vi "Shapelets Search (Brute Force).vi"() -> ()   [LabVIEW 2016]
uses:
  <vilib>/Math Plots/3D Math Plots/3D Ribbon/3D Ribbon XCtrl/3D Ribbon.xctl
  _vlib/SH_ApplicationStates.ctl
  _vlib/Shapelets Search Brute Force.lvclass
  _vlib/SH_Shapelet.ctl
  <vilib>/Math Plots/3D Math Plots/3D Ribbon/3D Ribbon Datatype/Public/Plot Helper (Standard).vi
  Shapelets Search (Brute Force).lvlib
  <vilib>/Math Plots/3D Math Plots/3D Ribbon/3D Ribbon Datatype/3D Ribbon Datatype.lvclass
panel:
  out "Progress Bar":i32(slide) caption="Ход выполнения" min=0 max=56 scale=0.0..18.0
  in  "Stop":bool
  out "Application State":string caption="Текущее состояние"
  in  "Tab Control":enum32{"Настройка поиска", "Результаты поиска"}(tab)
  out "Number of Training Trials":i32 caption="Всего записей в файле"
  out "Time series length":i32 caption="Длина каждой записи"
  in  "MinLength (in %)":dbl(slide)=0.2 caption="Мин. длина кандидата (в %)" min=0.0 max=1.0 step=0.05 scale=0.0..1.0
  in  "MaxLength (in %)":dbl(slide)=1.0 caption="Макс. длина кандидата (в %)" min=0.0 max=1.0 step=0.05 scale=0.0..1.0
  out "Number of Shapelets":i32 caption="Общее число кандидатов"
  in  "Enable pruning?":bool caption="Включить отбрасывание?"
  in  "Start Search":bool
  in  "Training Data":path caption="Путь к XML-файлу с исходными данными"
  in  "Number of Channels":i32=14 caption="Число каналов в записи"
  in  "Read File":bool
  in  "Save":bool
  out "Total num":i32
  in  "View":enum32{"3D вид", "2D вид"}(tab)
  out "3D Shapelet":refnum<class "3D Plot Datatype.lvclass">[](xcontrol) caption="3D вид шейплета"
  out "2D вид шейплета":cluster{i32[], dbl[]}[](graph)
  out "Fitness":dbl caption="Оценка качества" format="%#_3g"
  out "Shapelet Index":i32 caption="Номер кандидата"
  out "Shapelet Class":string caption="Метка класса"
  in  "Best Shapelets":i32(ring) caption="Список кандидатов в шейплеты" items=["42154"=42154, "38580"=38580, "40724"=40724, "40668"=40668, "39805"=39805, "40595"=40595, "38664"=38664, "31554"=31554, "41421"=41421, "42155"=42155, "42148"=42148, "41324"=41324, "37301"=37301, "42144"=42144, "41896"=41896, "41417"=41417, "39735"=39735, "29629"=29629, "26988"=26988, "26723"=26723, "12420"=12420, "41514"=41514, "41379"=41379, "40740"=40740, "39643"=39643, "37074"=37074, "35748"=35748, "33783"=33783, "18870"=18870, "18405"=18405, "42165"=42165, "42147"=42147, "41705"=41705, "39797"=39797, "38622"=38622, "37329"=37329, "27528"=27528, "27204"=27204, "21797"=21797, "15529"=15529, "11461"=11461, "42035"=42035, "41741"=41741, "41728"=41728, "41460"=41460, "41365"=41365, "41120"=41120, "38945"=38945, "38119"=38119, "36994"=36994, "35716"=35716, "35684"=35684, "35456"=35456, "35126"=35126, "33945"=33945, "33616"=33616, "32588"=32588, "31840"=31840, "31555"=31555, "29270"=29270, "26764"=26764, "24474"=24474, "24370"=24370, "11861"=11861]
  # "This VI is a part of BCI Design library, http://www.ru-bci.org \nCopyright © 2020, Sotnikov Peter, All rights reserved. License: GNU GPLv3"
  # "Исходные данные"
  # "Настройки поиска"
  # "Число рассматриваемых кандидатов:"
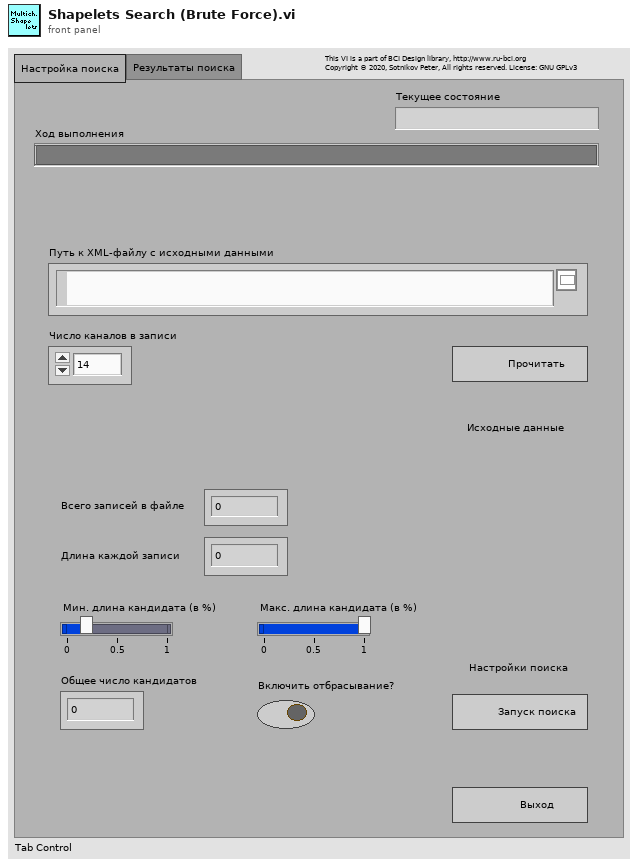
[diagram p1: front panel]
types:
  T1 = typedef "Shapelets Search (Brute Force).lvlib/SH_Shapelet.ctl" = cluster{"TrialIndex":i32, "Shift (in samples)":i32, "Length (in samples)":i32, "Distances":dbl[], "ClassIndecies":i32[], "Fitness":dbl, "Split Point":dbl}
  T2 = typedef "Shapelets Search (Brute Force).lvlib/SH_ApplicationStates.ctl" = enum16{"Start", "Read data", "Estimate  Number", "Generate Shapelets", "Find Best Shapelets", "Stop"}
  T3 = cluster{"Number of Training Trials":refnum<vi>, "Progress Bar":refnum<vi>}
  T4 = cluster{"Shapelet Index":refnum<vi>, "Fitness":refnum<vi>}
  T5 = typedef "LVStringsAndValuesArrayTypeDef_I32.ctl" = cluster{"String":string, "Value":i32}[]
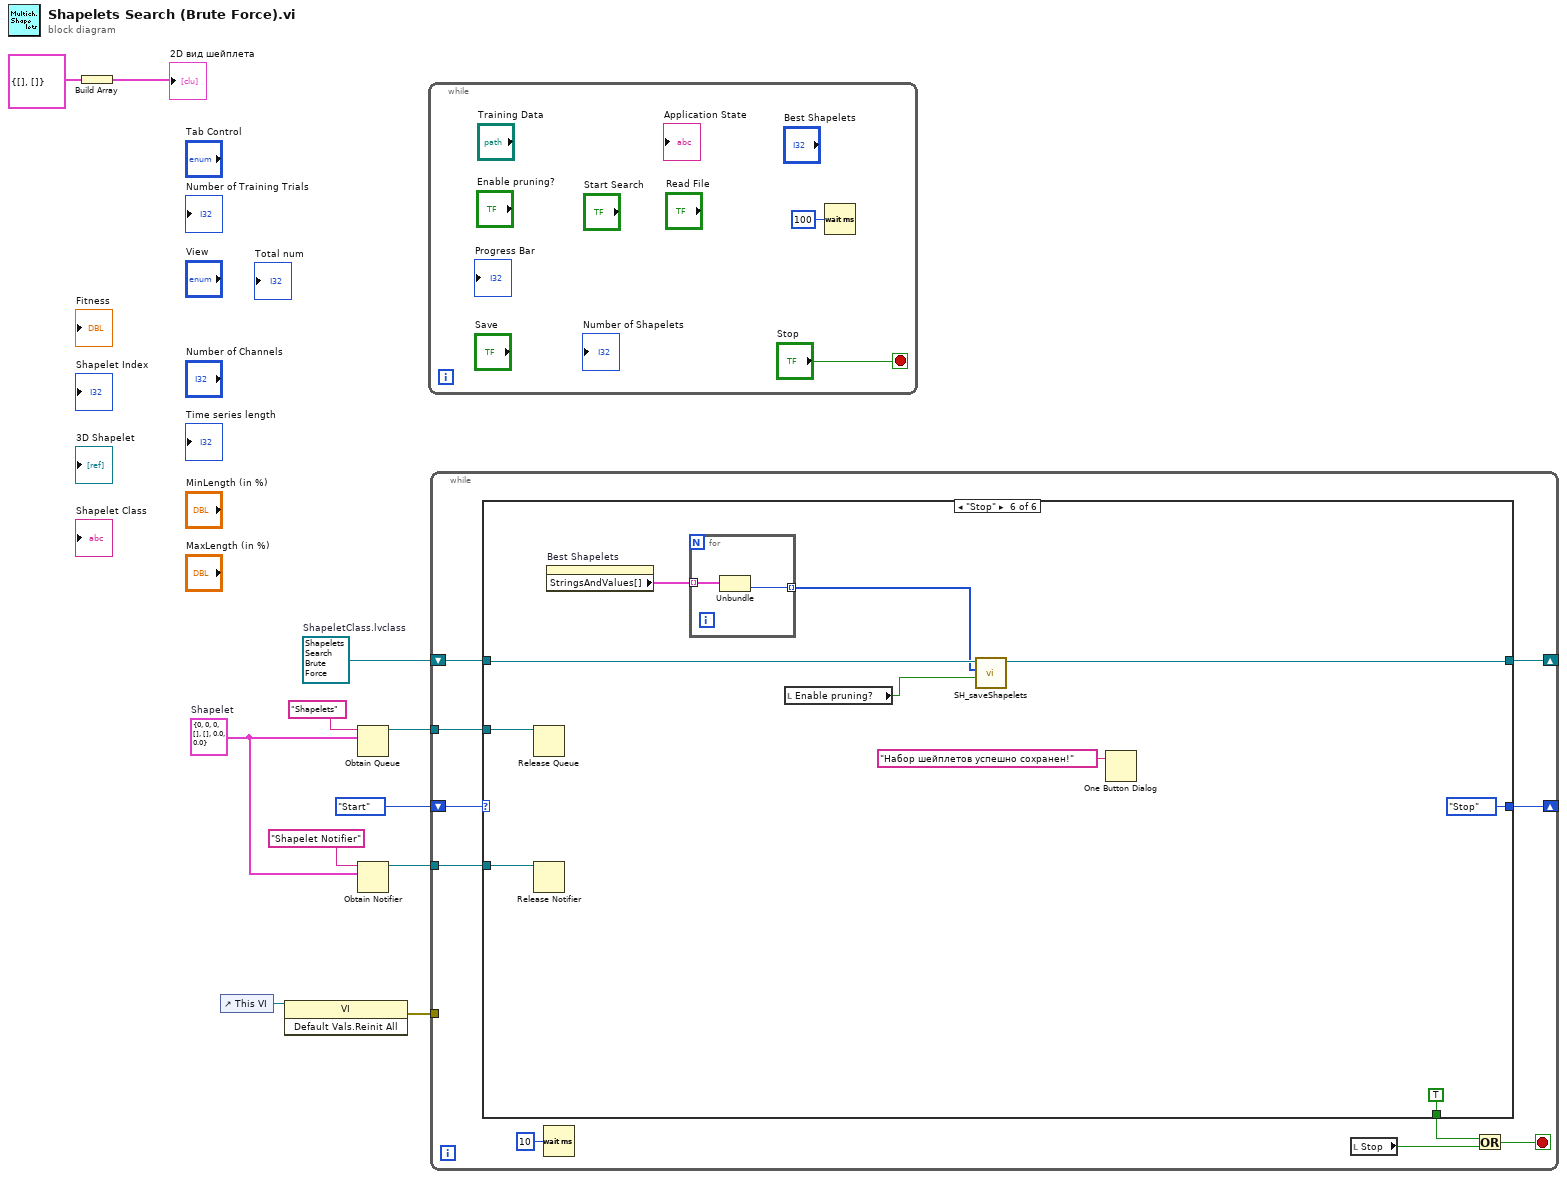
[diagram p0: block diagram]
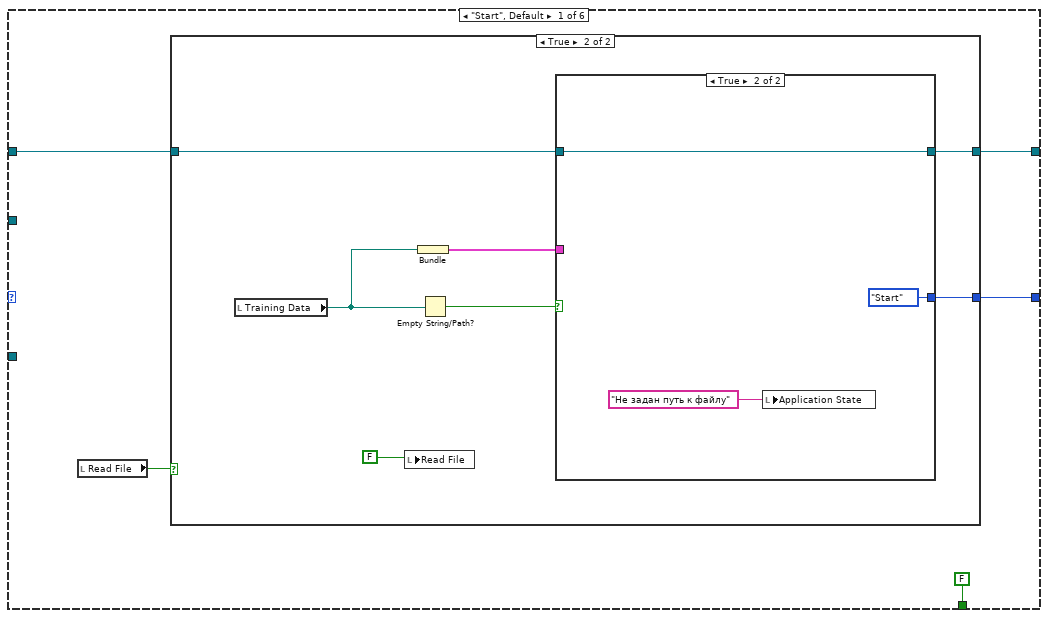
[diagram p2: hidden frame]
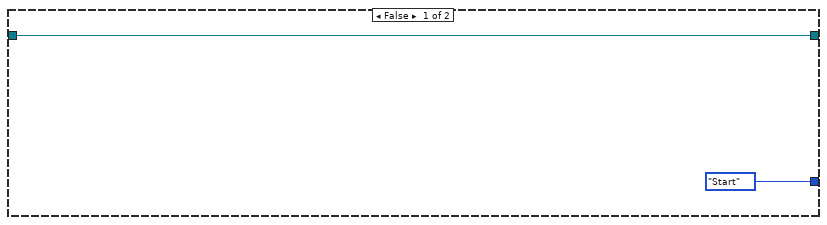
[diagram p3: hidden frame]
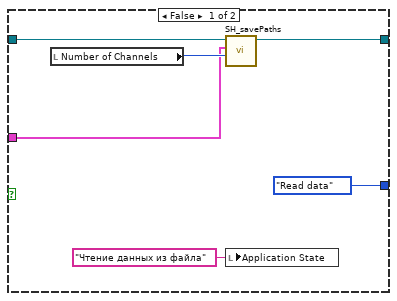
[diagram p4: hidden frame]
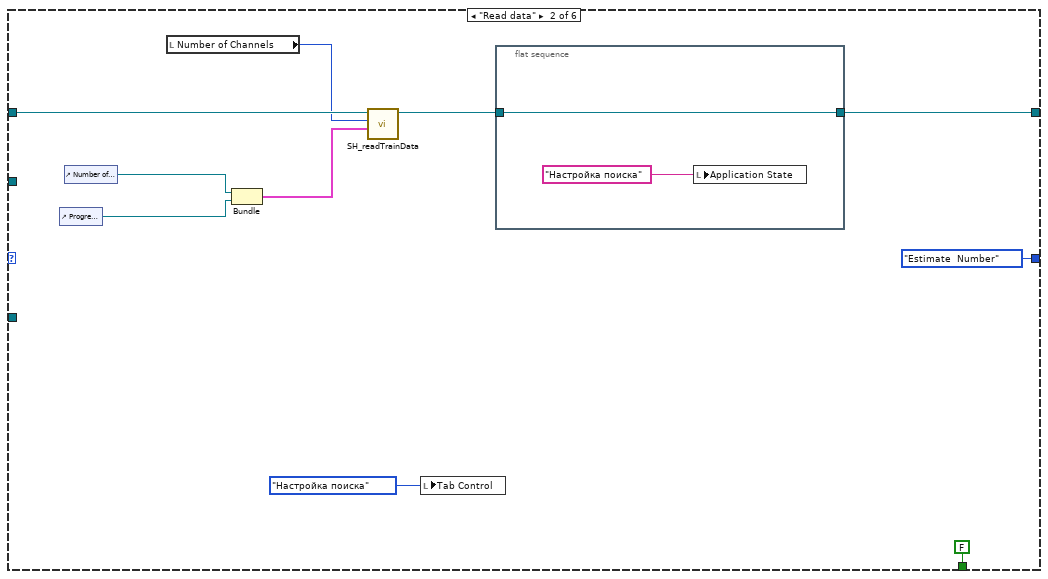
[diagram p5: hidden frame]
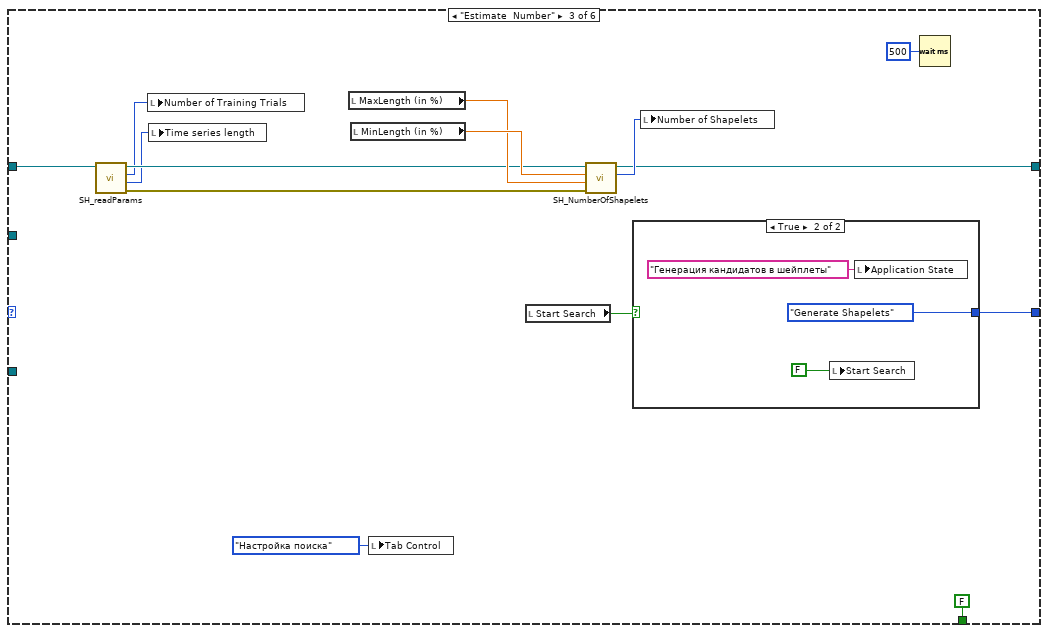
[diagram p6: hidden frame]
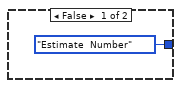
[diagram p7: hidden frame]
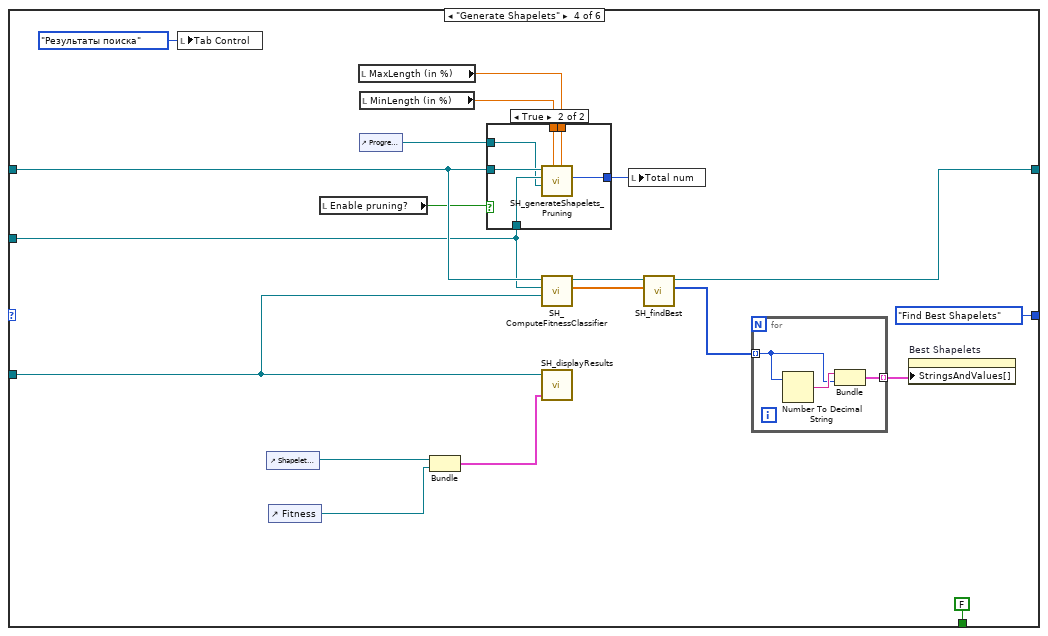
[diagram p8: hidden frame]
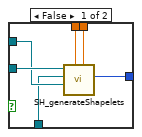
[diagram p9: hidden frame]
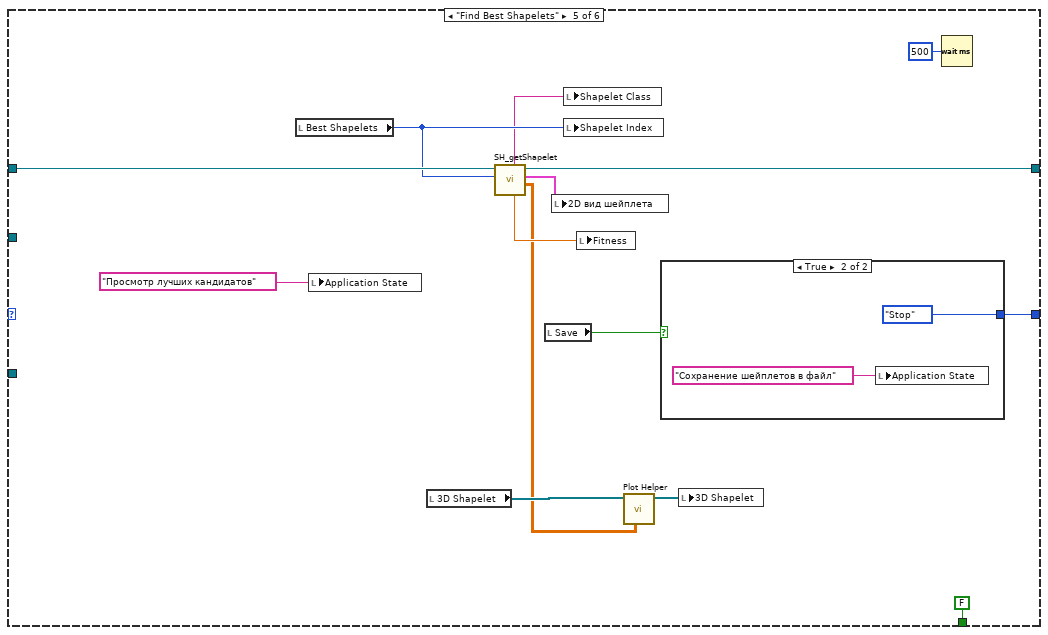
[diagram p10: hidden frame]
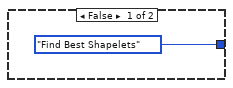
[diagram p11: hidden frame]
diagram:
  w4 = T1 {"TrialIndex"=0, "Shift (in samples)"=0, "Length (in samples)"=0, "Distances"=[], "ClassIndecies"=[], "Fitness"=0.0, "Split Point"=0.0}  # Shapelet
  w10 = refnum<class "Shapelets Search Brute Force.lvclass"> refnum  # ShapeletClass.lvclass
  n1 = Build Array(cluster{i32[], dbl[]} {[], []} ("Accuracy Chart")) -> (→"2D вид шейплета":cluster{i32[], dbl[]}[])
  n2 = control-ref of="This VI"() -> (w9:refnum<vi>)
  n3 = invoke class="VI" method="Default Vals.Reinit All"(reference=w9) -> (error out=w8:errorcluster)  [unwired: 2 in, 2 out]
  n4 = Obtain Queue(name (unnamed)="Shapelets", element data type=w4) -> (queue out=w7:refnum<queue>)  [unwired: 3 in, 2 out]
  n5 = Obtain Notifier(name (unnamed)="Shapelet Notifier", notification data type=w4) -> (notifier out=w3:refnum<notifier>)  [unwired: 2 in, 2 out]
  n6 = while {
    stop <- "Stop" stop-if-true
    n7 = Wait (ms)(milliseconds to wait=u32 100) -> ()  [unwired: 1 out]
  }
  n8 = while {
    shift-right: [w19] -> _
    shift-left: SH_ApplicationStates."Start" ("ApplicationStates") -> [w23]
    shift-right: [w16] -> _
    shift-left: w10 -> [w18]
    tunnel: w8 -> [_]
    tunnel: w7 -> [w15]
    tunnel: w3 -> [w14]
    stop <- w22 stop-if-true
    n9 = case shown="\"Stop\"" w23 {
      tunnel: [FALSE FALSE FALSE FALSE FALSE TRUE] -> w20
      tunnel: [w25 SH_ApplicationStates."Estimate  Number" ("ApplicationStates") w71 SH_ApplicationStates."Find Best Shapelets" ("ApplicationStates") w124 SH_ApplicationStates."Stop" ("ApplicationStates")] -> w19
      tunnel: w18 -> [w26 w56 w67 w93 w122 w132]
      tunnel: [w24 w47 w61 w82 w121 w130] -> w16
      tunnel: w15 -> [_ _ _ w84 _ w135]
      tunnel: w14 -> [_ _ _ w91 _ w134]
      frame "Start", Default {
        n10 = local read "Read File"() -> (w27:bool)
        n11 = case shown="True" w27 {
          tunnel: w26 -> [w29 w35]
          tunnel: [SH_ApplicationStates."Start" ("ApplicationStates") w36] -> w25
          tunnel: [w29 w34] -> w24
          frame False {
          }
          frame True {
            n12 = local read "Training Data"() -> (w37:path)
            n13 = local write "Read File"(FALSE ("Next")) -> ()
            n14 = Bundle("Training Data"=w37) -> (w33:cluster{"Training Data":path})  [unwired: 1 in]
            n15 = Empty String/Path?(string/path=w37) -> (empty?=w32:bool)
            n16 = case shown="True" w32 {
              tunnel: [SH_ApplicationStates."Read data" ("ApplicationStates") SH_ApplicationStates."Start" ("ApplicationStates")] -> w36
              tunnel: w35 -> [w42 w46]
              tunnel: [w41 w46] -> w34
              tunnel: w33 -> [w39 _]
              frame False {
                n17 = local read "Number of Channels"() -> (w40:i32)
                n18 = call "SH_savePaths.vi"("Number of Channels"=w40, "Paths"=w39, "ShapeletClass in"=w42) -> ("ShapeletClass out"=w41:refnum<class "Shapelets Search Brute Force.lvclass">)  [unwired: 7 in, 1 out]
                n19 = local write "Application State"("Чтение данных из файла" ("Application State")) -> ()
              }
              frame True {
                n20 = local write "Application State"("Не задан путь к файлу" ("Application State")) -> ()
              }
            }
          }
        }
      }
      frame "Read data" {
        n21 = control-ref of="Progress Bar"() -> (w49:refnum<vi>)
        n22 = control-ref of="Number of Training Trials"() -> (w54:refnum<vi>)
        n23 = local read "Number of Channels"() -> (w51:i32)
        n24 = Bundle("Number of Training Trials"=w54, "Progress Bar"=w49) -> (w53:T3)  [unwired: 1 in]
        n25 = call "SH_readTrainData.vi"("ControlRefs"=w53, "NumberOfChannels"=w51, "ShapeletClass in"=w56) -> ("ShapeletClass out"=w48:refnum<class "Shapelets Search Brute Force.lvclass">)  [unwired: 7 in, 1 out]
        n26 = local write "Tab Control"(enum32{"Настройка поиска", "Результаты поиска"}."Настройка поиска" ("Tab Control")) -> ()
        n27 = flat-sequence {
          tunnel: w48 -> [w58]
          tunnel: [w58] -> w47
          frame #0 {
            n28 = local write "Application State"("Настройка поиска" ("Application State")) -> ()
          }
        }
      }
      frame "Estimate  Number" {
        n29 = call-dynamic "SH_readParams.vi"("ShapeletClass in"=w67) -> ("error out"=w65:errorcluster, "FeatureVectorLength"=w63:i32, "NumberOfTrials"=w64:i32, "ShapeletClass out"=w66:refnum<class "Shapelets Search Brute Force.lvclass">)  [unwired: 7 in]
        n30 = local write "Number of Training Trials"(w64) -> ()
        n31 = local write "Time series length"(w63) -> ()
        n32 = local read "MaxLength (in %)"() -> (w69:dbl)
        n33 = local read "MinLength (in %)"() -> (w70:dbl)
        n34 = local write "Tab Control"(enum32{"Настройка поиска", "Результаты поиска"}."Настройка поиска" ("Tab Control")) -> ()
        n35 = local read "Start Search"() -> (w60:bool)
        n36 = call "SH_NumberOfShapelets.vi"("error in (no error)"=w65, "MaxLength (in %)"=w69, "MinLength (in %)"=w70, "ShapeletClass in"=w66) -> ("Number of Shapelets"=w68:i32, "ShapeletClass out"=w61:refnum<class "Shapelets Search Brute Force.lvclass">)  [unwired: 5 in, 1 out]
        n37 = case shown="True" w60 {
          tunnel: [SH_ApplicationStates."Estimate  Number" ("ApplicationStates") SH_ApplicationStates."Generate Shapelets" ("ApplicationStates")] -> w71
          frame False {
          }
          frame True {
            n38 = local write "Start Search"(FALSE ("Accept")) -> ()
            n39 = local write "Application State"("Генерация кандидатов в шейплеты" ("Application State")) -> ()
          }
        }
        n40 = local write "Number of Shapelets"(w68) -> ()
        n41 = Wait (ms)(milliseconds to wait=u32 500) -> ()  [unwired: 1 out]
      }
      frame "Generate Shapelets" {
        n42 = local write "Tab Control"(enum32{"Настройка поиска", "Результаты поиска"}."Результаты поиска" ("Tab Control")) -> ()
        n43 = control-ref of="Shapelet Index"() -> (w90:refnum<vi>)
        n44 = control-ref of="Fitness"() -> (w89:refnum<vi>)
        n45 = local read "Enable pruning?"() -> (w78:bool)
        n46 = local read "MaxLength (in %)"() -> (w86:dbl)
        n47 = local read "MinLength (in %)"() -> (w87:dbl)
        n48 = control-ref of="Progress Bar"() -> (w85:refnum<vi>)
        n49 = Bundle("Shapelet Index"=w90, "Fitness"=w89) -> (w88:T4)  [unwired: 1 in]
        n50 = case shown="True" w78 {
          tunnel: w93 -> [w101 w107]
          tunnel: [w100 w102] -> w92
          tunnel: w87 -> [w99 w106]
          tunnel: w86 -> [w98 w105]
          tunnel: w85 -> [w97 w103]
          tunnel: w84 -> [w96 w104]
          frame False {
            n51 = call "SH_generateShapelets.vi"("MaxLength (in %)"=w98, "MinLength (in %)"=w99, "Progress"=w97, "Shapelets Queue"=w96, "ShapeletClass in"=w101) -> ("Total Number of Shapelets"=w100:i32)  [unwired: 4 in, 2 out]
          }
          frame True {
            n52 = call "SH_generateShapelets_Pruning.vi"("MaxLength (in %)"=w105, "MinLength (in %)"=w106, "Progress"=w103, "Shapelets Queue"=w104, "ShapeletClass in"=w107) -> ("Total Number of Shapelets"=w102:i32)  [unwired: 4 in, 2 out]
          }
        }
        n53 = call "SH_ComputeFitnessClassifier.vi"("Notifier"=w91, "Shapelets Queue"=w84, "ShapeletClass in"=w93) -> ("Fitness Values"=w81:dbl[], "ShapeletClass out"=w83:refnum<class "Shapelets Search Brute Force.lvclass">)  [unwired: 6 in, 1 out]
        n54 = call "SH_displayResults.vi"("Control Refs"=w88, "Shapelet Notifier"=w91) -> ()  [unwired: 3 in]
        n55 = local write "Total num"(w92) -> ()
        n56 = call "SH_findBest.vi"("Fitness Values"=w81, "ShapeletClass in"=w83) -> ("Best Indicies"=w80:i32[], "ShapeletClass out"=w82:refnum<class "Shapelets Search Brute Force.lvclass">)  [unwired: 5 in]
        n57 = for {
          tunnel: w80 -> [w109] mode=indexing
          tunnel: [w108] -> w79 mode=indexing
          n58 = Number To Decimal String(number=w109) -> (decimal integer string=w110:string)  [unwired: 1 in]
          n59 = Bundle(w110, w109) -> (w108:cluster{string, i32})  [unwired: 1 in]
        }
        n60 = property on="Best Shapelets" class="Ring (strict)"("StringsAndValues[]"=w79) -> ()  [unwired: 2 in, 2 out]
      }
      frame "Find Best Shapelets" {
        n61 = local read "Best Shapelets"() -> (w118:i32)
        n62 = local write "Application State"("Просмотр лучших кандидатов" ("Application State")) -> ()
        n63 = local read "3D Shapelet"() -> (w115:refnum<class "3D Plot Datatype.lvclass">[])
        n64 = call "SH_getShapelet.vi"("Index"=w118, "ShapeletClass in"=w122) -> ("Shapelet"=w114:dbl[][], "ShapeletForm"=w120:cluster{i32[], dbl[]}[], "ShapeletClass out"=w121:refnum<class "Shapelets Search Brute Force.lvclass">, "Fitness"=w119:dbl, "ClassLabel"=w111:string)  [unwired: 4 in, 1 out]
        n65 = local read "Save"() -> (w116:bool)
        n66 = local write "2D вид шейплета"(w120) -> ()
        n67 = local write "Shapelet Class"(w111) -> ()
        n68 = local write "Shapelet Index"(w118) -> ()
        n69 = local write "Fitness"(w119) -> ()
        n70 = call-poly <vilib>:"Plot Helper.vi"("z matrix"=w114, "3D Plot lvclass Array in"=w115) -> ("3D Plot lvclass Array out"=w113:refnum<class "3D Plot Datatype.lvclass">[])  [unwired: 3 in, 6 out]
        n71 = case shown="True" w116 {
          tunnel: [SH_ApplicationStates."Find Best Shapelets" ("ApplicationStates") SH_ApplicationStates."Stop" ("ApplicationStates")] -> w124
          frame False {
          }
          frame True {
            n72 = local write "Application State"("Сохранение шейплетов в файл" ("Application State")) -> ()
          }
        }
        n73 = local write "3D Shapelet"(w113) -> ()
        n74 = Wait (ms)(milliseconds to wait=u32 500) -> ()  [unwired: 1 out]
      }
      frame "Stop" {
        n75 = Release Queue(queue=w135) -> ()  [unwired: 2 in, 3 out]
        n76 = Release Notifier(notifier=w134) -> ()  [unwired: 2 in, 3 out]
        n77 = property on="Best Shapelets" class="Ring (strict)"() -> ("StringsAndValues[]"=w133:T5)  [unwired: 2 in, 2 out]
        n78 = for {
          tunnel: w133 -> [w139] mode=indexing
          tunnel: [w138] -> w131 mode=indexing
          n79 = Unbundle(w139) -> ("Value"=w138:i32)  [unwired: 1 out]
        }
        n80 = local read "Enable pruning?"() -> (w129:bool)
        n81 = call "SH_saveShapelets.vi"("Pruning on?"=w129, "Indicies"=w131, "ShapeletClass in"=w132) -> ("ShapeletClass out"=w130:refnum<class "Shapelets Search Brute Force.lvclass">)  [unwired: 7 in, 1 out]
        n82 = One Button Dialog(message="Набор шейплетов успешно сохранен!") -> ()  [unwired: 1 in, 1 out]
      }
    }
    n83 = Wait (ms)(milliseconds to wait=u32 10) -> ()  [unwired: 1 out]
    n84 = local read "Stop"() -> (w21:bool)
    n85 = Or(x=w20, y=w21) -> (x .or. y?=w22:bool)
  }
